vi "get-conunt.vi"(10 "tool# or drive subsystem name":string, 11 "Tool array in":T1[](array[typedef])) -> (2 "Found?":bool, 3 "Count":i32)   [LabVIEW 2017, in "labview-standard-library.lvlib" / "automode-scripting.lvlib"]
uses:
  automode-scripting.lvlib
  type-defs/tool-call-tracker.ctl
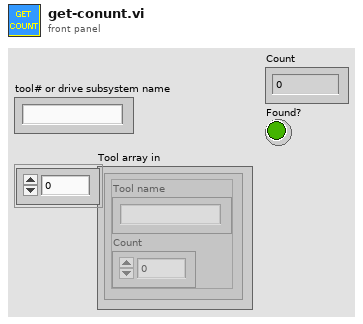
[diagram p1: front panel]
types:
  T1 = typedef "tool-call-tracker.ctl" = cluster{"Tool name":string, "Count":i32}
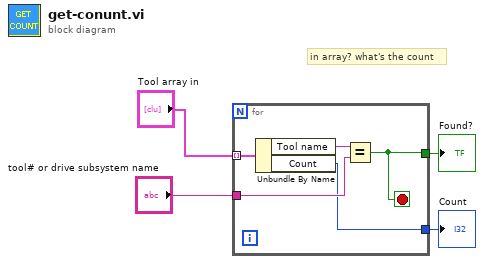
[diagram p0: block diagram]
diagram:
  # "in array? what's the count"
  n1 = for {
    tunnel: "Tool array in" -> [w9] mode=indexing
    tunnel: "tool# or drive subsystem name" -> [w7]
    tunnel: [w6] -> w1
    tunnel: [w5] -> w2
    stop <- w6 stop-if-true
    n2 = Unbundle By Name(w9) -> ("Tool name"=w8:string, "Count"=w5:i32)
    n3 = Equal?(x=w8, y=w7) -> (x = y?=w6:bool)
  }
  "Count" <- w2
  "Found?" <- w1
